vi "TestSquareRoot.vi"(11 "Error In":errorcluster) -> (15 "Error Out":errorcluster)   [LabVIEW 2016, in "SimpleCalculatorTests.lvlib"]
doc: "This VI is used for validating square root function"
uses:
  SimpleCalculatorTests.lvlib
  APIs/Stimulus/ControlValue/SetValueAuto.vi
  APIs/Stimulus/KeyBoardSimulation/KeyboardSimulationCore.vi
  APIs/Stimulus/VI/CloseVI.vi
  Drona.lvlib
  <vilib>/addons/_JKI Toolkits/Caraya/classes/Test/Test.lvclass
  <vilib>/SLL Toolkit/SLL Debug/SLL Debug.lvlib
  APIs/Stimulus/VI/VI.lvlib
  APIs/Stimulus/KeyBoardSimulation/KeyboardSimulation.lvlib
  APIs/Stimulus/ControlValue/ControlValue.lvlib
panel:
  # "Drona Test Square Root"
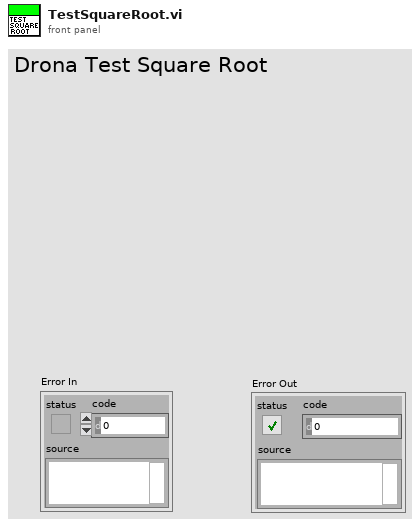
[diagram p1: front panel]
types:
  T1 = cluster{" Key":u8, "Action":enum16{"Press", "Up", "Down"}, "Delay (ms)":u32}[]
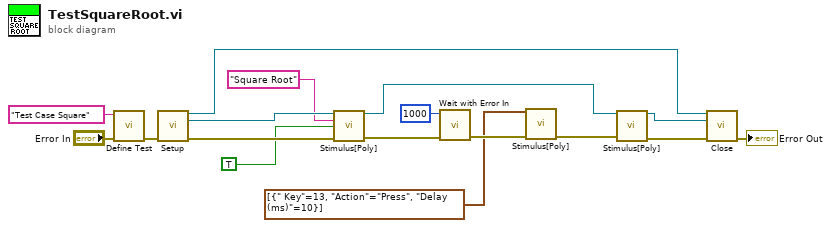
[diagram p0: block diagram]
diagram:
  n1 = call <vilib>:"Define Test.vi"("error in (no error)"="Error In", "Label (VI Title)"="Test Case Square") -> ("error out"=w17:errorcluster)  [unwired: 9 in]
  n2 = call "Setup.vi"("error in"=w17) -> ("Application Ref"=w2:refnum<vi>, "VI Reference Out"=w14:refnum<vi>, "error out"=w15:errorcluster)  [unwired: 12 in]
  n3 = call-poly "Stimulus[Poly].vi"("VI Reference In"=w14, "Control Path"="Square Root", "Value (Signaling)"=TRUE, "error in"=w15) -> ("VI Reference Out"=w4:refnum<vi>, "error out"=w11:errorcluster)  [unwired: 10 in]
  n4 = call <vilib>:"Wait with Error In.vi"("error in (no error)"=w11, "milliseconds to wait"=u32 1000) -> ("error out"=w9:errorcluster)  [unwired: 9 in]
  n5 = call-poly "Stimulus[Poly].vi"("Key Array"=T1 [{" Key"=13, "Action"=enum."Press", "Delay (ms)"=10}], "error in"=w9) -> ("error out"=w8:errorcluster)  [unwired: 13 in]
  n6 = call-poly "Stimulus[Poly].vi"("VI Reference In"=w4, "error in"=w8) -> ("VI Reference Out"=w3:refnum<vi>, "error out"=w5:errorcluster)  [unwired: 12 in]
  n7 = call "Close.vi"("Application Ref"=w2, "VI Reference"=w3, "error in"=w5) -> ("error out"=→"Error Out":errorcluster)  [unwired: 12 in]
